vi "Configure CRD Route Data.vi"(8 "error in":errorcluster, 10 "CfgRefIn":T1, 11 "Controller in":refnum<class "Controller.lvclass">) -> (0 "error out":errorcluster, 2 "CfgRefOut":T1, 3 "Controller out":refnum<class "Controller.lvclass">)   [LabVIEW 2014, in "Controller.lvlib" / "Controller.lvclass"]
doc: "This VI takes care of establishing proper routes for device data required for real-time CRD computation. The routing data is stored in variant attributes. The first tier of variant attributes contains:\n\n* IDs - this is a list of device IDs as defined in the configuration file.\n* Device ID - contains an associated variant which in turn contains an array for each variable P, T, and Q. The array contains the associated cell.\n\nThe variant is stored in a DVR which allows cross loop communication. This data which will be stored will be used to send regular update messages to the CRD for it's use."
uses:
  Controller.lvclass
  <vilib>/Utility/config.llb/Config Data RefNum.ctl
  Controller.lvclass/Controller.ctl
  <vilib>/Utility/config.llb/Read Key (I32).vi
  <vilib>/Utility/config.llb/Read Key (String).vi
  <vilib>/Utility/config.llb/NI_LVConfig.lvlib
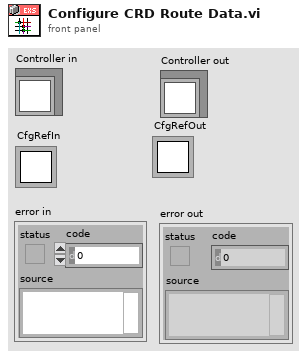
[diagram p1: front panel]
types:
  T1 = typedef "NI_LVConfig.lvlib/Config Data RefNum.ctl" = refnum<k1>
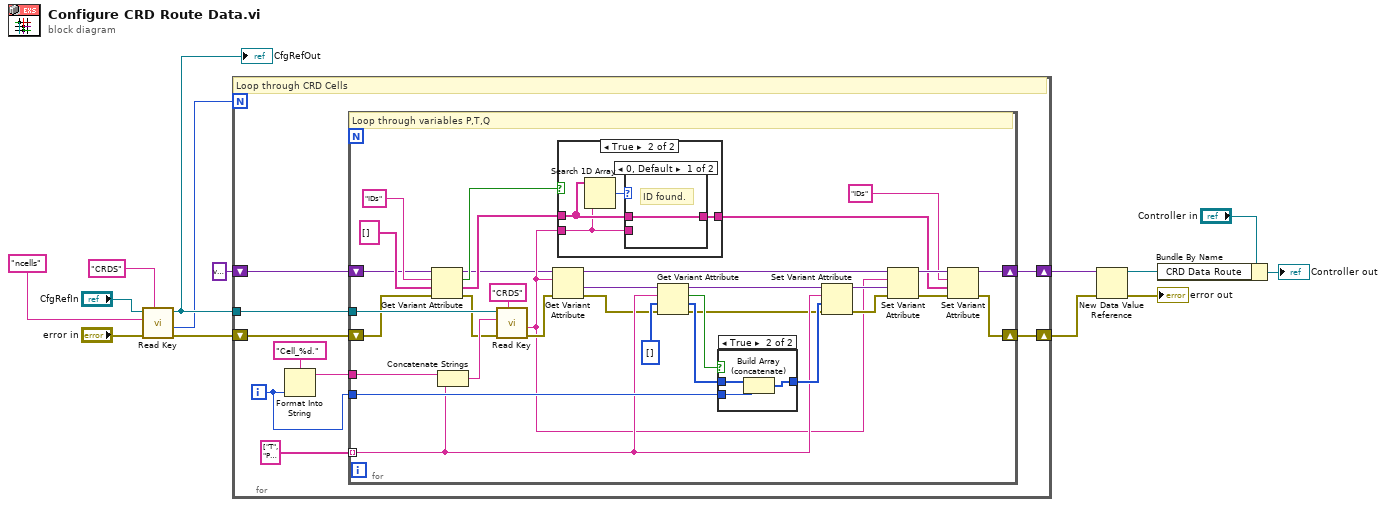
[diagram p0: block diagram]
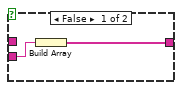
[diagram p2: hidden frame]
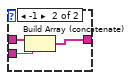
[diagram p3: hidden frame]
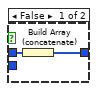
[diagram p4: hidden frame]
diagram:
  n1 = call-poly <vilib>:"Read Key.vi"("section"="CRDS", "error in (no error)"="error in", "key"="ncells", "refnum"="CfgRefIn") -> ("error out"=w8:errorcluster, "value"=w10:i32, "refnum out"=w12:T1)  [unwired: 4 in, 1 out]
  "CfgRefOut" <- w12
  n2 = for {
    N: w10 -> [_]
    tunnel: w12 -> [w23]
    shift-right: [w18] -> w4
    shift-left: variant -> [w19]
    shift-right: [w15] -> w2
    shift-left: w8 -> [w16]
    i -> [w17]
    # "Loop through CRD Cells"
    n3 = Format Into String(format string="Cell_%d.", w17) -> (resulting string=w21:string)  [unwired: 2 in, 1 out]
    n4 = for {
      tunnel: w23 -> [w56]
      tunnel: w21 -> [w55]
      tunnel: string[] ["T", "P", "Q"] -> [w47] mode=indexing
      shift-right: [w36] -> w18
      shift-left: w19 -> [w30]
      tunnel: w17 -> [w50]
      shift-right: [w34] -> w15
      shift-left: w16 -> [w28]
      # "Loop through variables P,T,Q"
      n5 = Get Variant Attribute(Variant=w30, name="IDs", default value (empty Variant)=string[] [], error in=w28) -> (duplicate Variant=w29:variant, found=w40:bool, value=w39:string[], error out=w27:errorcluster)
      n6 = Concatenate Strings(w55, w47) -> (w42:string)
      n7 = call-poly <vilib>:"Read Key.vi"("section"="CRDS", "error in (no error)"=w27, "key"=w42, "refnum"=w56) -> ("error out"=w45:errorcluster, "value"=w38:string)  [unwired: 4 in, 2 out]
      n8 = Get Variant Attribute(Variant=w29, name=w38, error in=w45) -> (duplicate Variant=w24:variant, value=w54:variant, error out=w25:errorcluster)  [unwired: 1 in, 1 out]
      n9 = case shown="True" w40 {
        tunnel: w39 -> [_ w61]
        tunnel: w38 -> [w58 w60]
        tunnel: [w57 w59] -> w32
        frame False {
          n10 = Build Array(w58) -> (w57:string[])
        }
        frame True {
          n11 = Search 1D Array(1D array=w61, element=w60) -> (index of element=w62:i32)  [unwired: 1 in]
          n12 = case shown="0, Default" w62 {
            tunnel: w61 -> [w63 w66]
            tunnel: w60 -> [_ w65]
            tunnel: [w63 w64] -> w59
            frame 0, Default {
              # "ID found."
            }
            frame -1 {
              n13 = Build Array (concatenate)(w66, w65) -> (w64:string[])
            }
          }
        }
      }
      n14 = Get Variant Attribute(Variant=w54, name=w47, default value (empty Variant)=i32[] [], error in=w25) -> (duplicate Variant=w48:variant, found=w52:bool, value=w51:i32[], error out=w44:errorcluster)
      n15 = case shown="True" w52 {
        tunnel: w51 -> [w68 w71]
        tunnel: w50 -> [_ w70]
        tunnel: [w67 w69] -> w49
        frame False {
          n16 = Build Array (concatenate)(w68) -> (w67:i32[])
        }
        frame True {
          n17 = Build Array (concatenate)(w71, w70) -> (w69:i32[])
        }
      }
      n18 = Set Variant Attribute(Variant=w48, name=w47, value=w49, error in=w44) -> (Variant out=w46:variant, error out=w43:errorcluster)  [unwired: 1 out]
      n19 = Set Variant Attribute(Variant=w24, name=w38, value=w46, error in=w43) -> (Variant out=w37:variant, error out=w35:errorcluster)  [unwired: 1 out]
      n20 = Set Variant Attribute(Variant=w37, name="IDs", value=w32, error in=w35) -> (Variant out=w36:variant, error out=w34:errorcluster)  [unwired: 1 out]
    }
  }
  n21 = New Data Value Reference(data value=w4, error in=w2) -> (data value reference=w3:refnum<data-value>, error out=→"error out":errorcluster)
  n22 = Bundle By Name(cluster="Controller in", "CRD Data Route"=w3) -> (→"Controller out":refnum<class "Controller.lvclass">)
